vi "SetSystemDefinitionFile.vi"(6 "path root vi ref (calling vi)":refnum<vi>, 8 "error in (no error)":errorcluster, 10 "system definition file":path, 11 "VeriStandTestCase in":refnum<class "VeriStandTestCase.lvclass">) -> (0 "error out":errorcluster, 3 "VeriStandTestCase out":refnum<class "VeriStandTestCase.lvclass">)   [LabVIEW 2016, in "VeriStandTestCase.lvclass"]
uses:
  VeriStandTestCase.lvclass
  VeriStandTestCase.lvclass/VeriStandTestCase.ctl
  VeriStandTestUtilities/VeriStandTestUtilities.lvlib
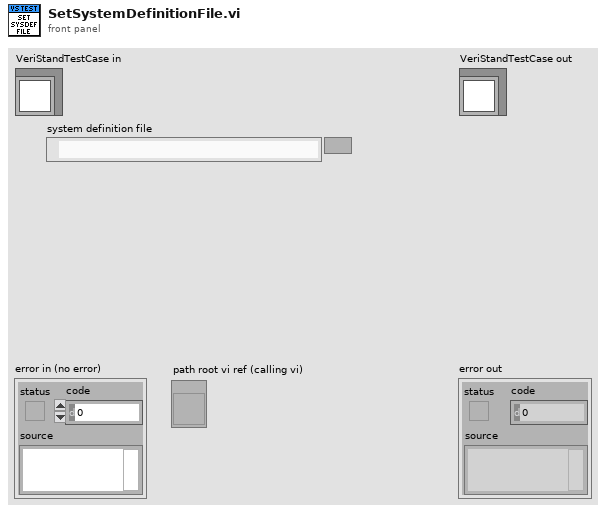
[diagram p1: front panel]
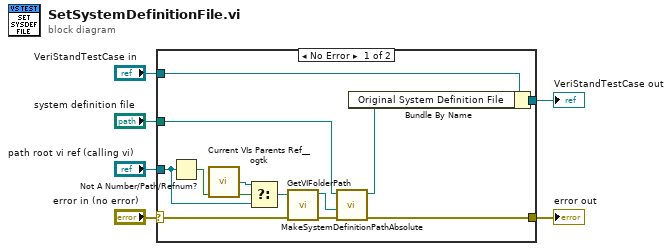
[diagram p0: block diagram]
diagram:
  n1 = case shown="No Error" "error in (no error)" {
    selector: "error in (no error)" -> [w18 w20]
    tunnel: [w10 w20] -> w5
    tunnel: [w12 w19] -> w3
    tunnel: "VeriStandTestCase in" -> [w13 w19]
    tunnel: "system definition file" -> [w8 _]
    tunnel: "path root vi ref (calling vi)" -> [w14 _]
    frame No Error {
      n2 = Not A Number/Path/Refnum?(number/path/refnum=w14) -> (NaN/Path/Refnum?=w17:bool)
      n3 = call <userlib>:"Current VIs Parents Ref__ogtk.vi"() -> ("Calling VI's Reference"=w16:refnum<vi>)  [unwired: 2 in]
      n4 = Select(t=w16, s=w17, f=w14) -> (s? t:f=w15:refnum<vi>)
      n5 = call "GetVIFolderPath.vi"("error in (no error)"=w18, "VI Reference in"=w15) -> ("error out"=w11:errorcluster, "VI Folder Path out"=w7:path)  [unwired: 8 in]
      n6 = call "MakeSystemDefinitionPathAbsolute.vi"("error in (no error)"=w11, "relative base path"=w7, "system definition file"=w8) -> ("error out"=w10:errorcluster, "absolute system definition file"=w9:path)  [unwired: 7 in]
      n7 = Bundle By Name(cluster=w13, "Original System Definition File"=w9) -> (w12:refnum<class "VeriStandTestCase.lvclass">)
    }
    frame Error {
    }
  }
  "error out" <- w5
  "VeriStandTestCase out" <- w3
